vi "IPI_AutoTest.vi"() -> ()   [LabVIEW 2015]
uses:
  <vilib>/Utility/file.llb/Read Delimited Spreadsheet (string).vi
panel:
  out "Version Param Out":string[][](array[string])=[["3;0;3;1;39.700;4;0;1;0;0;1;65280;255;16776960;16711680;", "3;0;5;1;44.800;4;0;1;0;0;1;65280;255;16776960;16711680;", "3;0;7;1;51.000;4;0;1;0;0;1;65280;255;16776960;16711680;", "3;0;15;7;33.000;4;0;1;0;0;1;65280;255;16776960;16711680;", "Null", "Null", "Null", "Null", "Null"], ["3;0;5;1;91.000;4;0;1;0;0;1;65280;255;16776960;16711680;", "2;2;5;1;30.000;4;0;1;0;0;1;65280;255;16776960;16711680;", "3;2;55;29;72.900;4;0;1;0;0;1;65280;255;16776960;16711680;", "Null", "Null", "Null", "Null", "Null", "Null"], ["3;0;5;1;104.000;4;0;1;0;0;1;65280;255;16776960;16711680;", "2;2;7;1;74.000;4;0;1;0;0;1;65280;255;16776960;16711680;", "3;2;25;9;63.600;4;0;1;0;0;1;65280;255;16776960;16711680;", "Null", "Null", "Null", "Null", "Null", "Null"], ["3;0;5;1;44.200;4;0;1;0;0;1;65280;255;16776960;16711680;", "2;0;5;1;63.400;4;0;1;0;0;1;65280;255;16776960;16711680;", "3;0;13;1;95.200;4;0;1;0;0;1;65280;255;16776960;16711680;", "Null", "Null", "Null", "Null", "Null", "Null"], ["3;0;5;1;102.000;4;0;1;0;0;1;65280;255;16776960;16711680;", "2;0;7;1;62.000;4;0;1;0;0;1;65280;255;16776960;16711680;", "3;2;29;33;55.000;4;0;1;0;0;1;65280;255;16776960;16711680;", "Null", "Null", "Null", "Null", "Null", "Null"], ["3;0;5;1;53.700;4;0;1;0;0;1;65280;255;16776960;16711680;", "2;2;7;1;70.000;4;0;1;0;0;1;65280;255;16776960;16711680;", "3;2;5;3;73.100;4;0;1;0;0;1;65280;255;16776960;16711680;", "Null", "Null", "Null", "Null", "Null", "Null"], ["3;0;5;1;109.000;4;0;1;0;0;1;65280;255;16776960;16711680;", "2;2;3;9;34.000;4;0;1;0;0;1;65280;255;16776960;16711680;", "3;2;5;1;30.200;4;0;1;0;0;1;65280;255;16776960;16711680;", "Null", "Null", "Null", "Null", "Null", "Null"], ["3;0;5;1;72.000;4;0;1;0;0;1;65280;255;16776960;16711680;", "3;2;7;1;38.500;4;0;1;0;0;1;65280;255;16776960;16711680;", "2;2;7;1;84.000;4;0;1;0;0;1;65280;255;16776960;16711680;", "3;2;9;1;41.500;4;0;1;0;0;1;65280;255;16776960;16711680;", "Null", "Null", "Null", "Null", "Null"], ["3;0;5;1;58.700;4;0;1;0;0;1;65280;255;16776960;16711680;", "2;2;11;1;45.000;4;0;1;0;0;1;65280;255;16776960;16711680;", "3;2;27;13;73.500;4;0;1;0;0;1;65280;255;16776960;16711680;", "Null", "Null", "Null", "Null", "Null", "Null"]] caption="Vision Params"
  in  "等待时间（毫秒）":u32=10
  out "路径 2":path
  out "Image":T1(plugin-control)
  in  "字符串":string="Snap16.tiff"
  out "All Files in Dir":path[](array[path]) caption="目录中的所有文件"
  in  "路径":path=path "C:/DataPicture/20160702"
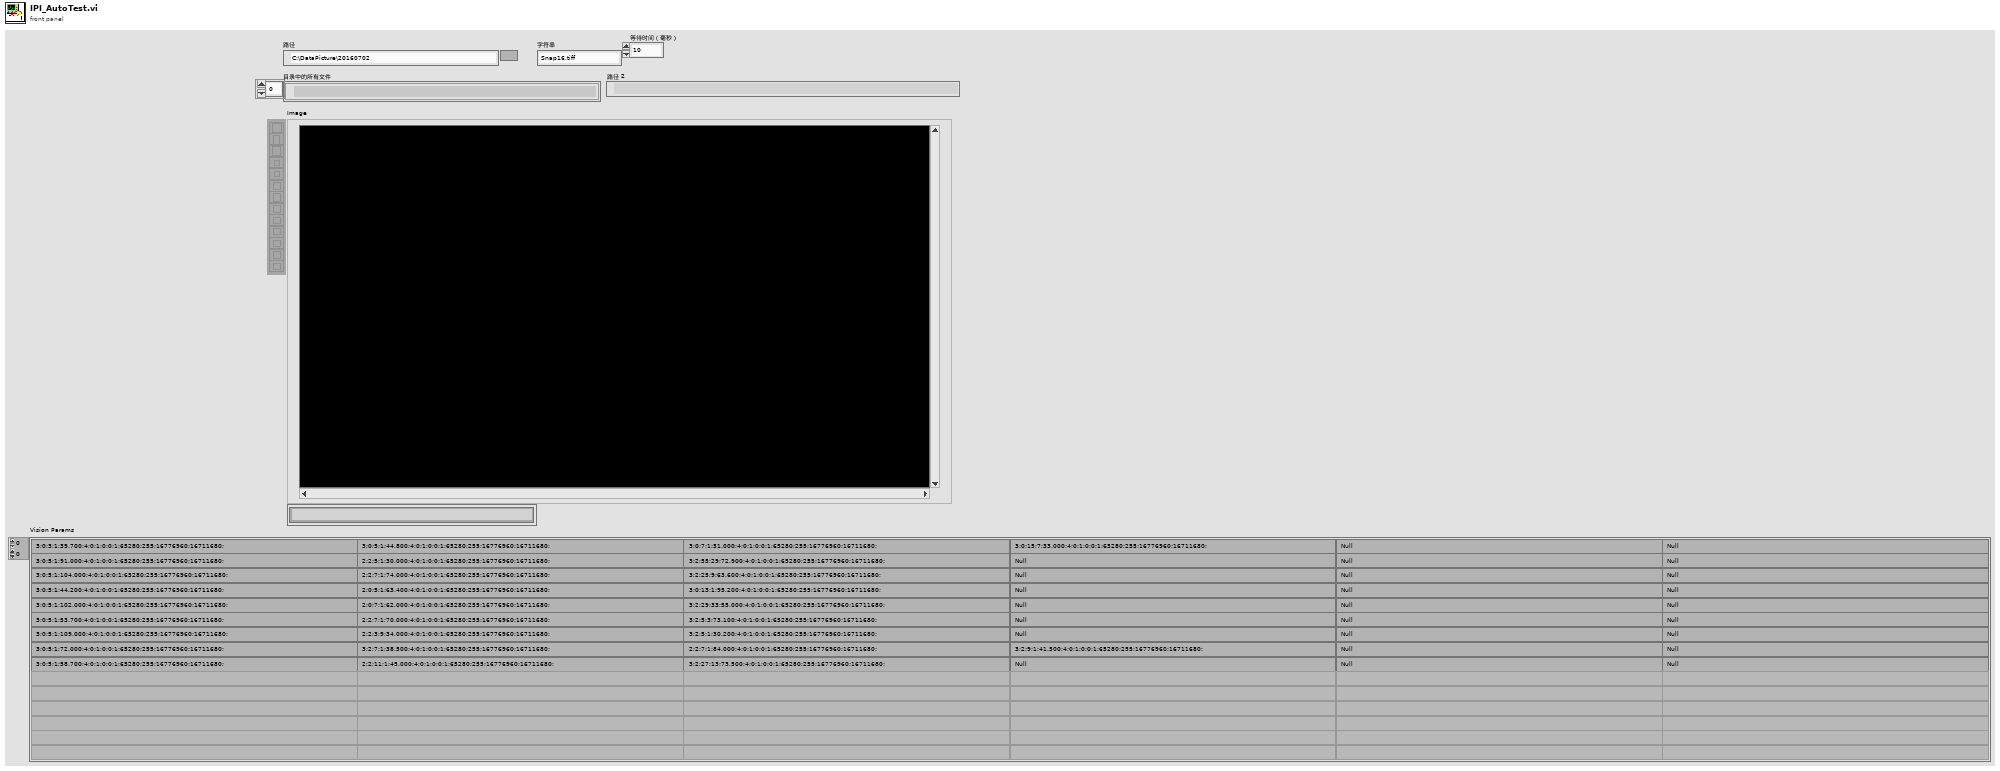
[diagram p1: front panel]
types:
  T1 = typedef "IMAQ Image.ctl" = refnum<image>
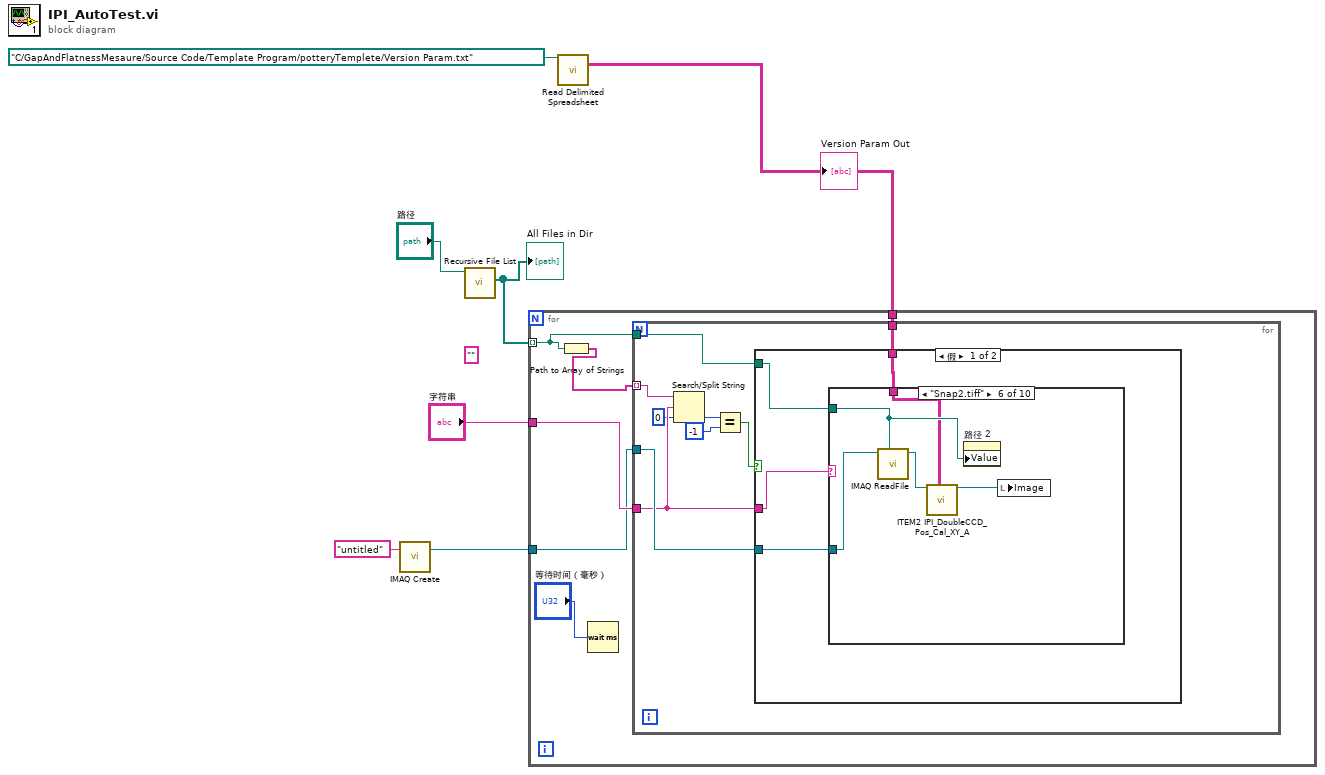
[diagram p0: block diagram]
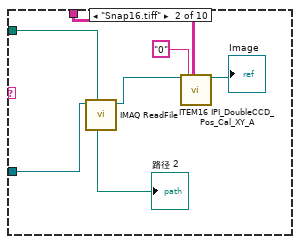
[diagram p3: hidden frame]
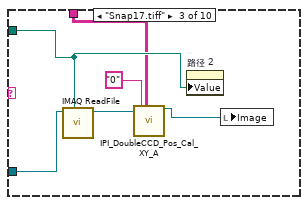
[diagram p4: hidden frame]
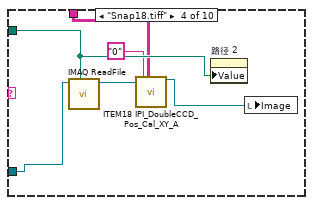
[diagram p5: hidden frame]
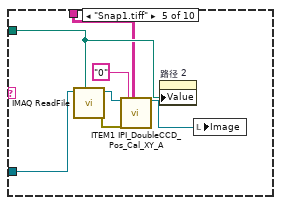
[diagram p6: hidden frame]
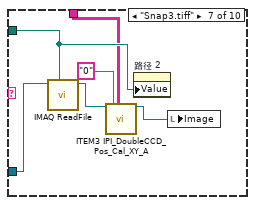
[diagram p7: hidden frame]
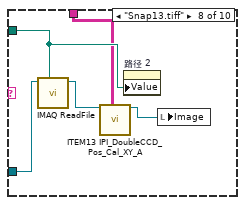
[diagram p8: hidden frame]
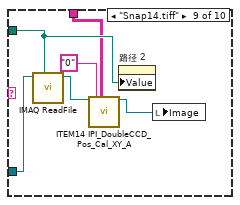
[diagram p9: hidden frame]
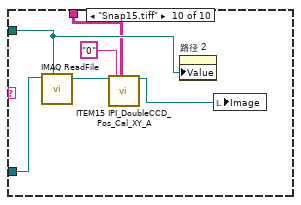
[diagram p10: hidden frame]
diagram:
  (unwired) ""
  n1 = call "IMAQ Create"("Image Name"="untitled") -> ("New Image"=w3:T1)  [unwired: 4 in, 1 out]
  n2 = call <vilib>:"Recursive File List.vi"("Folder Path"="路径") -> ("All Files in Dir"=w6:path[])  [unwired: 6 in, 4 out]
  "All Files in Dir" <- w6
  n3 = call-poly <vilib>:"Read Delimited Spreadsheet.vi"("file path (dialog if empty)"=path "C:/GapAndFlatnessMesaure/Source Code/Template Program/potteryTemplete/Version Param.txt") -> ("all rows"=w1:string[][])  [unwired: 9 in, 5 out]
  "Version Param Out" <- w1
  n4 = for {
    tunnel: w6 -> [w13] mode=indexing
    tunnel: "字符串" -> [w12]
    tunnel: w3 -> [w11]
    tunnel: w1 -> [w8]
    n5 = Path to Array of Strings(0:w13) -> (2:w10:string[])  [unwired: 1 out]
    n6 = Wait (ms)(milliseconds to wait="等待时间（毫秒）") -> ()  [unwired: 1 out]
    n7 = for {
      tunnel: w13 -> [w22]
      tunnel: w12 -> [w19]
      tunnel: w11 -> [w21]
      tunnel: w10 -> [w20] mode=indexing
      tunnel: w8 -> [w14]
      n8 = Search/Split String(string=w20, search string/char (-)=w19, offset (0)=0 ("偏移量(0)")) -> (offset of match=w17:i32)  [unwired: 2 out]
      n9 = Equal?(x=w17, y=-1) -> (x = y?=w15:bool)
      n10 = case shown="假" w15 {
        tunnel: w22 -> [w26 _]
        tunnel: w19 -> [w25 _]
        tunnel: w21 -> [w24 _]
        tunnel: w14 -> [w23 _]
        frame False {
          n11 = case shown="\"Snap2.tiff\"" w25 {
            tunnel: w26 -> [_ w31 w34 w41 w46 w55 w58 w64 w69 w75]
            tunnel: w24 -> [_ w32 w38 w44 w51 w56 w62 w67 w73 w79]
            tunnel: w23 -> [_ w27 w33 w39 w45 w52 w57 w63 w68 w74]
            frame "假", Default {
            }
            frame "Snap16.tiff" {
              n12 = call "IMAQ ReadFile"("File Path"=w31, "Image"=w32) -> ("Image Out"=w30:T1)  [unwired: 5 in, 4 out]
              n13 = call "ITEM16 IPI_DoubleCCD_Pos_Cal_XY_A.vi"("Image In"=w30, "offset"="0", "Version Param Out"=w27) -> ("Image"=→"Image":T1)  [unwired: 10 in, 6 out]
              "路径 2" <- w31
            }
            frame "Snap17.tiff" {
              n14 = call "IMAQ ReadFile"("File Path"=w34, "Image"=w38) -> ("Image Out"=w37:T1)  [unwired: 5 in, 4 out]
              n15 = call "IPI_DoubleCCD_Pos_Cal_XY_A.vi"("Image In"=w37, "offset"="0", "Version Param Out"=w33) -> ("Image"=w35:T1)  [unwired: 11 in, 5 out]
              n16 = property on="路径 2" class="Path"("Value"=w34) -> ()  [unwired: 2 in, 2 out]
              n17 = local write "Image"(w35) -> ()
            }
            frame "Snap18.tiff" {
              n18 = call "IMAQ ReadFile"("File Path"=w41, "Image"=w44) -> ("Image Out"=w43:T1)  [unwired: 5 in, 4 out]
              n19 = call "ITEM18 IPI_DoubleCCD_Pos_Cal_XY_A.vi"("Image In"=w43, "offset"="0", "Version Param Out"=w39) -> ("Image"=w42:T1)  [unwired: 12 in, 4 out]
              n20 = property on="路径 2" class="Path"("Value"=w41) -> ()  [unwired: 2 in, 2 out]
              n21 = local write "Image"(w42) -> ()
            }
            frame "Snap1.tiff" {
              n22 = call "IMAQ ReadFile"("File Path"=w46, "Image"=w51) -> ("error out"=w49:errorcluster, "Image Out"=w50:T1)  [unwired: 5 in, 3 out]
              n23 = call "ITEM1 IPI_DoubleCCD_Pos_Cal_XY_A.vi"("Image In"=w50, "error in"=w49, "offset"="0", "Version Param Out"=w45) -> ("Image"=w47:T1)  [unwired: 11 in, 4 out]
              n24 = property on="路径 2" class="Path"("Value"=w46) -> ()  [unwired: 2 in, 2 out]
              n25 = local write "Image"(w47) -> ()
            }
            frame "Snap2.tiff" {
              n26 = call "IMAQ ReadFile"("File Path"=w55, "Image"=w56) -> ("Image Out"=w54:T1)  [unwired: 5 in, 4 out]
              n27 = call "ITEM2 IPI_DoubleCCD_Pos_Cal_XY_A.vi"("Image In"=w54, "Version Param Out"=w52) -> ("Image"=w53:T1)  [unwired: 12 in, 5 out]
              n28 = property on="路径 2" class="Path"("Value"=w55) -> ()  [unwired: 2 in, 2 out]
              n29 = local write "Image"(w53) -> ()
            }
            frame "Snap3.tiff" {
              n30 = call "IMAQ ReadFile"("File Path"=w58, "Image"=w62) -> ("Image Out"=w61:T1)  [unwired: 5 in, 4 out]
              n31 = call "ITEM3 IPI_DoubleCCD_Pos_Cal_XY_A.vi"("Image In"=w61, "offset"="0", "Version Param Out"=w57) -> ("Image"=w59:T1)  [unwired: 12 in, 4 out]
              n32 = property on="路径 2" class="Path"("Value"=w58) -> ()  [unwired: 2 in, 2 out]
              n33 = local write "Image"(w59) -> ()
            }
            frame "Snap13.tiff" {
              n34 = call "IMAQ ReadFile"("File Path"=w64, "Image"=w67) -> ("Image Out"=w66:T1)  [unwired: 5 in, 4 out]
              n35 = call "ITEM13 IPI_DoubleCCD_Pos_Cal_XY_A.vi"("Image In"=w66, "Version Param Out"=w63) -> ("Image"=w65:T1)  [unwired: 12 in, 5 out]
              n36 = property on="路径 2" class="Path"("Value"=w64) -> ()  [unwired: 2 in, 2 out]
              n37 = local write "Image"(w65) -> ()
            }
            frame "Snap14.tiff" {
              n38 = call "IMAQ ReadFile"("File Path"=w69, "Image"=w73) -> ("Image Out"=w72:T1)  [unwired: 5 in, 4 out]
              n39 = call "ITEM14 IPI_DoubleCCD_Pos_Cal_XY_A.vi"("Image In"=w72, "offset"="0", "Version Param Out"=w68) -> ("Image"=w70:T1)  [unwired: 12 in, 4 out]
              n40 = property on="路径 2" class="Path"("Value"=w69) -> ()  [unwired: 2 in, 2 out]
              n41 = local write "Image"(w70) -> ()
            }
            frame "Snap15.tiff" {
              n42 = call "IMAQ ReadFile"("File Path"=w75, "Image"=w79) -> ("Image Out"=w78:T1)  [unwired: 5 in, 4 out]
              n43 = call "ITEM15 IPI_DoubleCCD_Pos_Cal_XY_A.vi"("Image In"=w78, "offset"="0", "Version Param Out"=w74) -> ("Image"=w76:T1)  [unwired: 11 in, 5 out]
              n44 = property on="路径 2" class="Path"("Value"=w75) -> ()  [unwired: 2 in, 2 out]
              n45 = local write "Image"(w76) -> ()
            }
          }
        }
        frame True {
        }
      }
    }
  }
